vi "UID.vi"(7 "Actor in":refnum<class "Actor.lvclass">) -> (2 "UID":i32)   [LabVIEW 2020, in "jettl.lvlib" / "Read Parent Attributes.lvlib"]
uses:
  Read Parent Attributes.lvlib
  Actor/Actor.lvclass
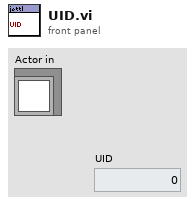
[diagram p1: front panel]
types:
  T1 = typedef "jettl.lvlib/Actor Attributes.ctl" = cluster{"Unified Layer":T2, "Root":bool, "Alias":string, "Transport":refnum<class "Transport.lvclass">, "UID":i32, "This VI":refnum<vi>, "Post-Setup Layers":refnum<class "Actor.lvclass">[]}
  T2 = typedef "jettl.lvlib/Unified Layer.ctl" = cluster{"Msgs":T3, "Leaf":bool}
  T3 = typedef "jettl.lvlib/Msgs.ctl" = set{refnum<class "Msg.lvclass">}
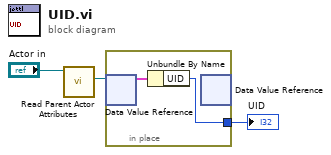
[diagram p0: block diagram]
diagram:
  n1 = call-dynamic "Read Parent Actor Attributes.vi"("Actor in"="Actor in") -> ("Parent Attributes"=w3:refnum<data-value>)  [unwired: 10 in]
  n2 = in-place {
    in-place-border: [w4] -> w1
    n3 = in-place-dvr #1(w3) -> (w5:T1)  [unwired: 1 out]
    n4 = Unbundle By Name(w5) -> ("UID"=w4:i32)
    n5 = in-place-dvr #1() -> ()  [unwired: 1 in, 2 out]
  }
  "UID" <- w1
